vi "getVideoFrame.vi"(6 "Frame increment":i32, 8 "error in (no error)":errorcluster, 9 "Start Frame Number":u32, 10 "Video fps":u32, 11 "Input cluster":T1) -> (0 "error out":errorcluster, 2 "Actual frame":u32, 3 "Output cluster":T1)   [LabVIEW 2020]
doc: "Get one frame from a video"
uses:
  controls/StateMachineVariables.ctl
  <vilib>/vision/Avi.llb/IMAQ AVI2 Refnum.ctl
  <vilib>/userDefined/High Color/IMAQdx.ctl
  <vilib>/vision/Deep Learning.llb/IMAQ DL Model Refnum.ctl
  <vilib>/vision/Image Controls.llb/IMAQ Image.ctl
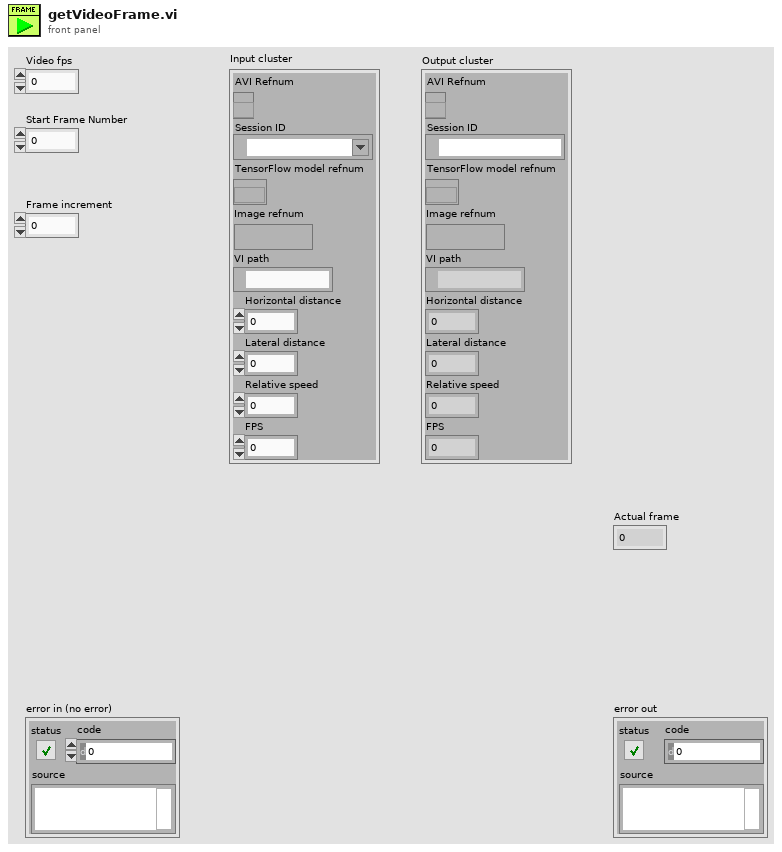
[diagram p1: front panel]
types:
  T1 = typedef "StateMachineVariables.ctl" = cluster{"AVI Refnum":T2, "Session ID":T3, "TensorFlow model refnum":T4, "Image refnum":T5, "VI path":path, "Horizontal distance":dbl, "Lateral distance":dbl, "Relative speed":dbl, "FPS":dbl}
  T2 = typedef "IMAQ AVI2 Refnum.ctl" = refnum<k20>
  T3 = typedef "IMAQdx.ctl" = refnum<k21>
  T4 = typedef "IMAQ DL Model Refnum.ctl" = refnum<k20>
  T5 = typedef "IMAQ Image.ctl" = refnum<image>
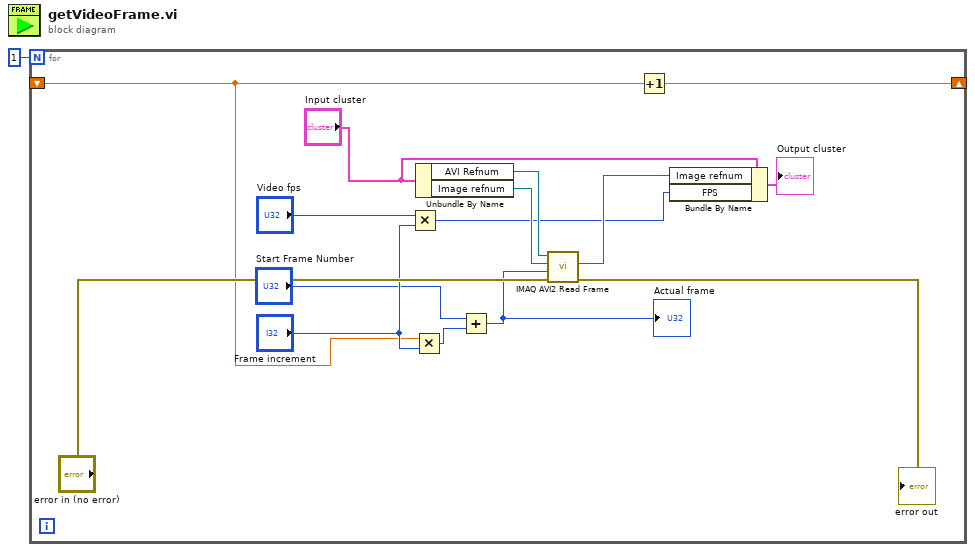
[diagram p0: block diagram]
diagram:
  n1 = for {
    N: 1 -> [_]
    shift-right: [w7] -> _
    shift-left: _ -> [w6]
    n2 = Multiply(x="Video fps", y="Frame increment") -> (x*y=w2:u32)
    n3 = Multiply(x=w6, y="Frame increment") -> (x*y=w8:i32)
    n4 = Unbundle By Name("Input cluster") -> ("AVI Refnum"=w14:T2, "Image refnum"=w15:T5)
    n5 = Add(x="Start Frame Number", y=w8) -> (x+y=w12:u32)
    "Actual frame" <- w12
    n6 = call "IMAQ AVI2 Read Frame"("error in (no error)"="error in (no error)", "Frame Number"=w12, "Image"=w15, "AVI Refnum"=w14) -> ("error out"=→"error out":errorcluster, "Image Out"=w5:T5)  [unwired: 5 in, 1 out]
    n7 = Increment(x=w6) -> (x+1=w7:dbl)
    n8 = Bundle By Name(cluster="Input cluster", "Image refnum"=w5, "FPS"=w2) -> (→"Output cluster":T1)
  }
